vi "ConvertIntArrayToBoolArray4x8.vi"(7 "intMatrix4x8":i32[][](array[numeric])) -> (8 "avgOut":bool[][](array[boolean]))   [LabVIEW 2016]
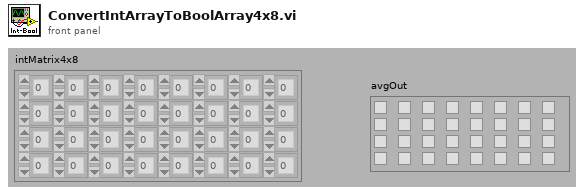
[diagram p1: front panel]
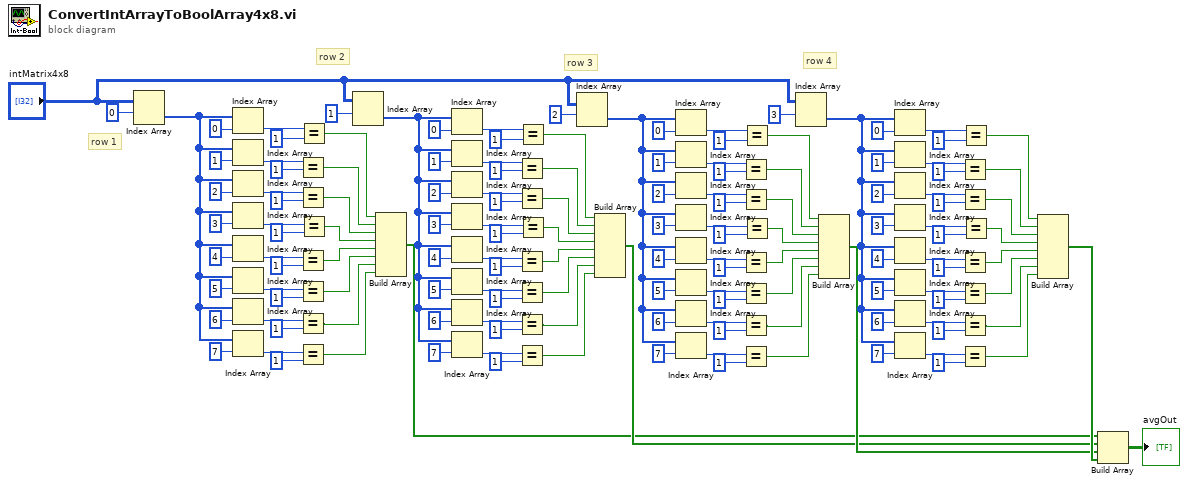
[diagram p0: block diagram]
diagram:
  # "row 4"
  # "row 3"
  # "row 2"
  # "row 1"
  n1 = Index Array(array="intMatrix4x8", index (row)=0) -> (element=w131:i32[])  [unwired: 1 in]
  n2 = Index Array(array=w131, index=0) -> (element=w139:i32)
  n3 = Index Array(array=w131, index=1) -> (element=w128:i32)
  n4 = Index Array(array=w131, index=2) -> (element=w126:i32)
  n5 = Index Array(array=w131, index=3) -> (element=w124:i32)
  n6 = Index Array(array=w131, index=4) -> (element=w122:i32)
  n7 = Index Array(array=w131, index=5) -> (element=w120:i32)
  n8 = Index Array(array=w131, index=6) -> (element=w118:i32)
  n9 = Index Array(array=w131, index=7) -> (element=w116:i32)
  n10 = Equal?(x=w128, y=1) -> (x = y?=w114:bool)
  n11 = Equal?(x=w126, y=1) -> (x = y?=w113:bool)
  n12 = Equal?(x=w122, y=1) -> (x = y?=w111:bool)
  n13 = Equal?(x=w120, y=1) -> (x = y?=w110:bool)
  n14 = Equal?(x=w118, y=1) -> (x = y?=w109:bool)
  n15 = Equal?(x=w116, y=1) -> (x = y?=w108:bool)
  n16 = Equal?(x=w139, y=1) -> (x = y?=w130:bool)
  n17 = Equal?(x=w124, y=1) -> (x = y?=w112:bool)
  n18 = Index Array(array="intMatrix4x8", index (row)=1) -> (element=w85:i32[])  [unwired: 1 in]
  n19 = Build Array(w130, w114, w113, w112, w111, w110, w109, w108) -> (w1:bool[])
  n20 = Index Array(array=w85, index=0) -> (element=w77:i32)
  n21 = Index Array(array=w85, index=1) -> (element=w87:i32)
  n22 = Index Array(array=w85, index=2) -> (element=w89:i32)
  n23 = Index Array(array=w85, index=3) -> (element=w91:i32)
  n24 = Index Array(array=w85, index=4) -> (element=w93:i32)
  n25 = Index Array(array=w85, index=5) -> (element=w95:i32)
  n26 = Index Array(array=w85, index=6) -> (element=w97:i32)
  n27 = Index Array(array=w85, index=7) -> (element=w99:i32)
  n28 = Equal?(x=w87, y=1) -> (x = y?=w101:bool)
  n29 = Equal?(x=w89, y=1) -> (x = y?=w102:bool)
  n30 = Equal?(x=w93, y=1) -> (x = y?=w104:bool)
  n31 = Equal?(x=w95, y=1) -> (x = y?=w105:bool)
  n32 = Equal?(x=w97, y=1) -> (x = y?=w106:bool)
  n33 = Equal?(x=w99, y=1) -> (x = y?=w107:bool)
  n34 = Equal?(x=w77, y=1) -> (x = y?=w86:bool)
  n35 = Equal?(x=w91, y=1) -> (x = y?=w103:bool)
  n36 = Index Array(array="intMatrix4x8", index (row)=2) -> (element=w62:i32[])  [unwired: 1 in]
  n37 = Build Array(w86, w101, w102, w103, w104, w105, w106, w107) -> (w2:bool[])
  n38 = Index Array(array=w62, index=0) -> (element=w70:i32)
  n39 = Index Array(array=w62, index=1) -> (element=w60:i32)
  n40 = Index Array(array=w62, index=2) -> (element=w58:i32)
  n41 = Index Array(array=w62, index=3) -> (element=w56:i32)
  n42 = Index Array(array=w62, index=4) -> (element=w54:i32)
  n43 = Index Array(array=w62, index=5) -> (element=w52:i32)
  n44 = Index Array(array=w62, index=6) -> (element=w50:i32)
  n45 = Index Array(array=w62, index=7) -> (element=w48:i32)
  n46 = Equal?(x=w60, y=1) -> (x = y?=w46:bool)
  n47 = Equal?(x=w58, y=1) -> (x = y?=w45:bool)
  n48 = Equal?(x=w54, y=1) -> (x = y?=w43:bool)
  n49 = Equal?(x=w52, y=1) -> (x = y?=w42:bool)
  n50 = Equal?(x=w50, y=1) -> (x = y?=w41:bool)
  n51 = Equal?(x=w48, y=1) -> (x = y?=w40:bool)
  n52 = Equal?(x=w70, y=1) -> (x = y?=w61:bool)
  n53 = Equal?(x=w56, y=1) -> (x = y?=w44:bool)
  n54 = Index Array(array="intMatrix4x8", index (row)=3) -> (element=w17:i32[])  [unwired: 1 in]
  n55 = Build Array(w61, w46, w45, w44, w43, w42, w41, w40) -> (w3:bool[])
  n56 = Index Array(array=w17, index=0) -> (element=w9:i32)
  n57 = Index Array(array=w17, index=1) -> (element=w19:i32)
  n58 = Index Array(array=w17, index=2) -> (element=w21:i32)
  n59 = Index Array(array=w17, index=3) -> (element=w23:i32)
  n60 = Index Array(array=w17, index=4) -> (element=w25:i32)
  n61 = Index Array(array=w17, index=5) -> (element=w27:i32)
  n62 = Index Array(array=w17, index=6) -> (element=w29:i32)
  n63 = Index Array(array=w17, index=7) -> (element=w31:i32)
  n64 = Equal?(x=w19, y=1) -> (x = y?=w33:bool)
  n65 = Equal?(x=w21, y=1) -> (x = y?=w34:bool)
  n66 = Equal?(x=w25, y=1) -> (x = y?=w36:bool)
  n67 = Equal?(x=w27, y=1) -> (x = y?=w37:bool)
  n68 = Equal?(x=w29, y=1) -> (x = y?=w38:bool)
  n69 = Equal?(x=w31, y=1) -> (x = y?=w39:bool)
  n70 = Equal?(x=w9, y=1) -> (x = y?=w18:bool)
  n71 = Equal?(x=w23, y=1) -> (x = y?=w35:bool)
  n72 = Build Array(w18, w33, w34, w35, w36, w37, w38, w39) -> (w4:bool[])
  n73 = Build Array(w1, w2, w3, w4) -> (→"avgOut":bool[][])
